vi "PCert-Application-Directories.vi"(11 "error in":errorcluster) -> (4 "Deploy Root":path, 6 "Provider Root":path, 15 "error out":errorcluster)   [LabVIEW 2013, in "PCert-ConfigPageNF.lvclass"]
uses:
  PCert-Container/ERP-ConfigPageNewFeather/PCert-ConfigPageNF.lvclass
panel:
  # "Inputs"
  # "Outputs"
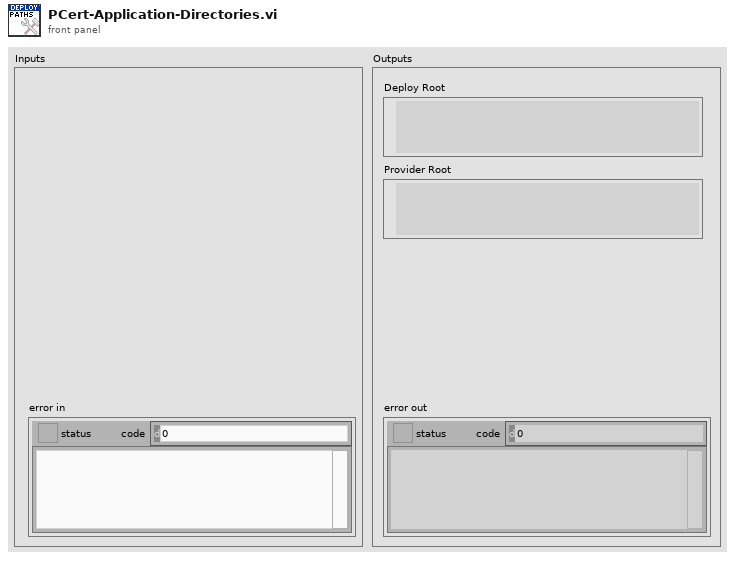
[diagram p1: front panel]
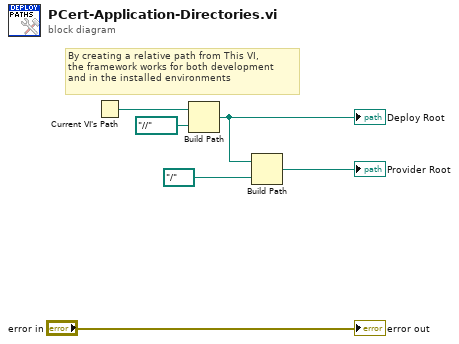
[diagram p0: block diagram]
diagram:
  # "By creating a relative path from This VI,\nthe framework works for both development\nand in the installed environments"
  n1 = Current VI's Path() -> (path=w6:path)
  n2 = Build Path(base path=w6, name or relative path=path "../../..") -> (appended path=w3:path)
  "Deploy Root" <- w3
  n3 = Build Path(base path=w3, name or relative path=path "../..") -> (appended path=→"Provider Root":path)
  "error out" <- "error in"
